vi "Fade Out.vi"(8 "error in (no error)":errorcluster, 11 "Rectangle Mask in":refnum<class "Rectangle Mask.lvclass">) -> (0 "error out":errorcluster, 3 "Rectangle Mask out":refnum<class "Rectangle Mask.lvclass">)   [LabVIEW 2016, in "Rectangle Mask.lvclass"]
uses:
  Rectangle Mask.lvclass
  Rectangle Mask.lvclass/Rectangle Mask.ctl
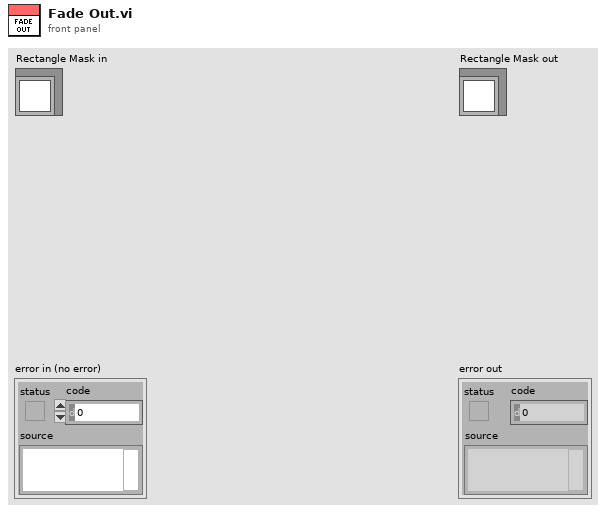
[diagram p1: front panel]
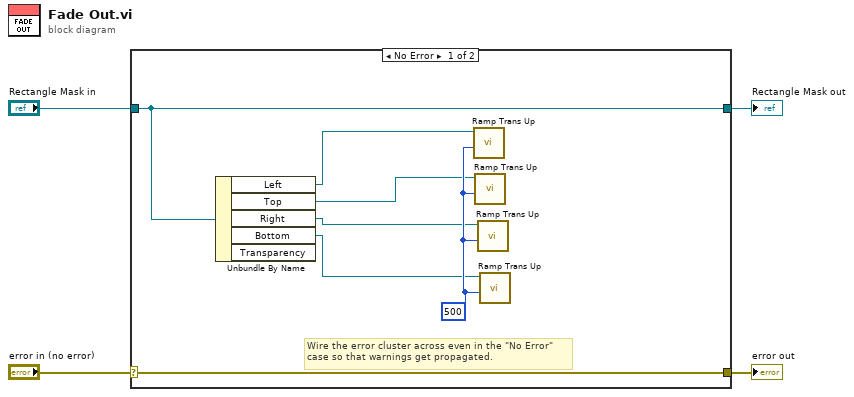
[diagram p0: block diagram]
diagram:
  n1 = case shown="No Error" "error in (no error)" {
    selector: "error in (no error)" -> [w11 w13]
    tunnel: [w11 w13] -> w3
    tunnel: [w5 w12] -> w1
    tunnel: "Rectangle Mask in" -> [w5 w12]
    frame No Error {
      w10 = u32 500 ("Time (ms)")
      # "Wire the error cluster across even in the \"No Error\"\ncase so that warnings get propagated."
      n2 = Unbundle By Name(w5) -> ("Left"=w9:refnum<vi>, "Top"=w8:refnum<vi>, "Right"=w7:refnum<vi>, "Bottom"=w6:refnum<vi>)  [unwired: 1 out]
      n3 = call "Ramp Trans Up.vi"("Time (ms)"=w10, "VI Ref In"=w9) -> ()  [unwired: 10 in]
      n4 = call "Ramp Trans Up.vi"("Time (ms)"=w10, "VI Ref In"=w8) -> ()  [unwired: 10 in]
      n5 = call "Ramp Trans Up.vi"("Time (ms)"=w10, "VI Ref In"=w7) -> ()  [unwired: 10 in]
      n6 = call "Ramp Trans Up.vi"("Time (ms)"=w10, "VI Ref In"=w6) -> ()  [unwired: 10 in]
    }
    frame Error {
    }
  }
  "error out" <- w3
  "Rectangle Mask out" <- w1
